vi "Attitude Control Open.vi"(10 "Scene Graph":refnum<vi>) -> (0 "error out":errorcluster, 3 "Attitude Control Handle":T1)   [LabVIEW 2015, in "lv-attitudecontrol.lvlib"]
uses:
  lv-attitudecontrol.lvlib
  Controls/AttitudeHandle.ctl
  <vilib>/picture/3D Picture Control/NI_3D Picture Control.lvlib
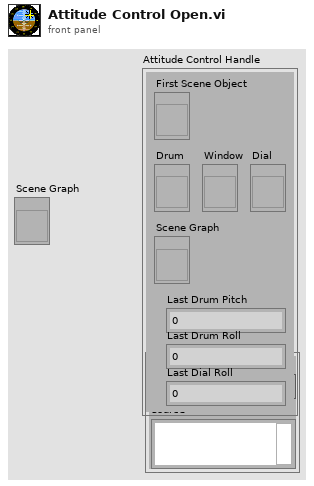
[diagram p1: front panel]
types:
  T1 = typedef "lv-attitudecontrol.lvlib/AttitudeHandle.ctl" = cluster{"First Scene Object":refnum<vi>, "Drum":refnum<vi>, "Window":refnum<vi>, "Dial":refnum<vi>, "Scene Graph":refnum<vi>, "Last Drum Pitch":dbl, "Last Drum Roll ":dbl, "Last Dial Roll":dbl}
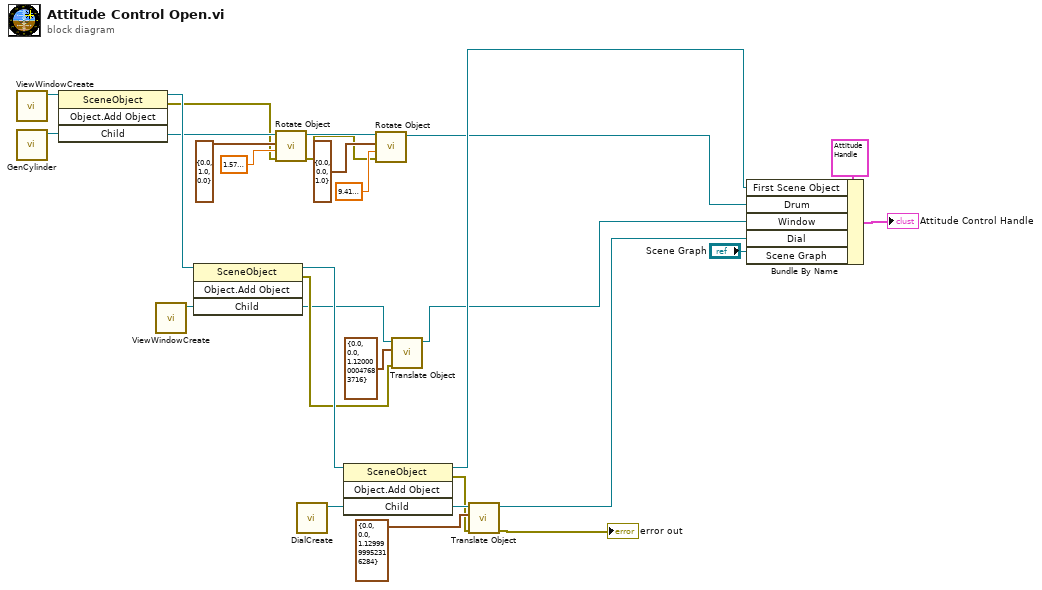
[diagram p0: block diagram]
diagram:
  n1 = call "ViewWindowCreate.vi"() -> ("SceneObject out"=w27:refnum<vi>)  [unwired: 11 in]
  n2 = call "GenCylinder.vi"() -> ("SceneObject out"=w18:refnum<vi>)  [unwired: 11 in]
  n3 = invoke class="SceneObject" method="Object.Add Object"(reference=w27, "Child"=w18) -> (reference out=w26:refnum<vi>, error out=w10:errorcluster, "Child"=w22:refnum<vi>)  [unwired: 2 in, 1 out]
  n4 = call "ViewWindowCreate.vi"() -> ("SceneObject out"=w28:refnum<vi>)  [unwired: 11 in]
  n5 = invoke class="SceneObject" method="Object.Add Object"(reference=w26, "Child"=w28) -> (reference out=w17:refnum<vi>, error out=w8:errorcluster, "Child"=w2:refnum<vi>)  [unwired: 2 in, 1 out]
  n6 = call <vilib>:"Rotate Object.vi"("error in (no error)"=w10, "Angle"=sgl 1.5799999 ("Angle 2"), "Axis"=cluster{"X":sgl, "Y":sgl, "Z":sgl} {"X"=0.0, "Y"=1.0, "Z"=0.0} ("Axis 2"), "Scene.Object In"=w22) -> ("error out"=w9:errorcluster, "Scene.Object Out"=w23:refnum<vi>)  [unwired: 6 in]
  n7 = call "DialCreate.vi"() -> ("SceneObject out"=w4:refnum<vi>)  [unwired: 11 in]
  n8 = invoke class="SceneObject" method="Object.Add Object"(reference=w17, "Child"=w4) -> (reference out=w15:refnum<vi>, error out=w3:errorcluster, "Child"=w6:refnum<vi>)  [unwired: 2 in, 1 out]
  n9 = call <vilib>:"Rotate Object.vi"("error in (no error)"=w9, "Angle"=sgl 9.419999 ("Angle 3"), "Axis"=cluster{"X":sgl, "Y":sgl, "Z":sgl} {"X"=0.0, "Y"=0.0, "Z"=1.0} ("Axis 3"), "Scene.Object In"=w23) -> ("Scene.Object Out"=w14:refnum<vi>)  [unwired: 6 in, 1 out]
  n10 = call <vilib>:"Translate Object.vi"("error in (no error)"=w8, "Translation"=cluster{"X":sgl, "Y":sgl, "Z":sgl} {"X"=0.0, "Y"=0.0, "Z"=1.12} ("Translation 4"), "Scene.Object In"=w2) -> ("Scene.Object Out"=w1:refnum<vi>)  [unwired: 7 in, 1 out]
  n11 = call <vilib>:"Translate Object.vi"("error in (no error)"=w3, "Translation"=cluster{"X":sgl, "Y":sgl, "Z":sgl} {"X"=0.0, "Y"=0.0, "Z"=1.13} ("Translation 5"), "Scene.Object In"=w6) -> ("error out"=→"error out":errorcluster, "Scene.Object Out"=w13:refnum<vi>)  [unwired: 7 in]
  n12 = Bundle By Name(cluster=T1 {"First Scene Object"=refnum, "Drum"=refnum, "Window"=refnum, "Dial"=refnum, "Scene Graph"=refnum, "Last Drum Pitch"=0.0, "Last Drum Roll "=0.0, "Last Dial Roll"=0.0} ("Attitude Control Handle"), "First Scene Object"=w15, "Drum"=w14, "Window"=w1, "Dial"=w13, "Scene Graph"="Scene Graph") -> (→"Attitude Control Handle":T1)
